vi "Divide XY (multiple).vi"(8 "error in (no error)":errorcluster, 9 "y":cluster{"X-array":dbl[], "Y-array":dbl[]}, 11 "XY-data":cluster{"X-array":dbl[], "Y-array":dbl[]}[](array[cluster]) {"Y-array" format="%.2p"; "X-array" format="%.2p"}) -> (0 "error out":errorcluster, 3 "XY-data out":cluster{"X-array":dbl[], "Y-array":dbl[]}[](array[cluster]) {"Y-array" format="%.2p"; "X-array" format="%.2p"})   [LabVIEW 2019, in "xy_utilities.lvlib"]
doc: "Divide <b>y</b>'s y array by the y array of <b>XY-data</b>.\n\nWire data to the data input to determine the polymorphic instance to use or manually select the instance."
uses:
  xy_utilities.lvlib
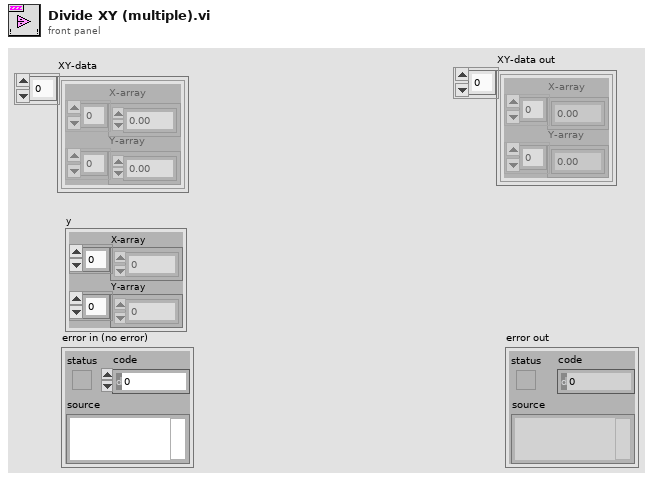
[diagram p1: front panel]
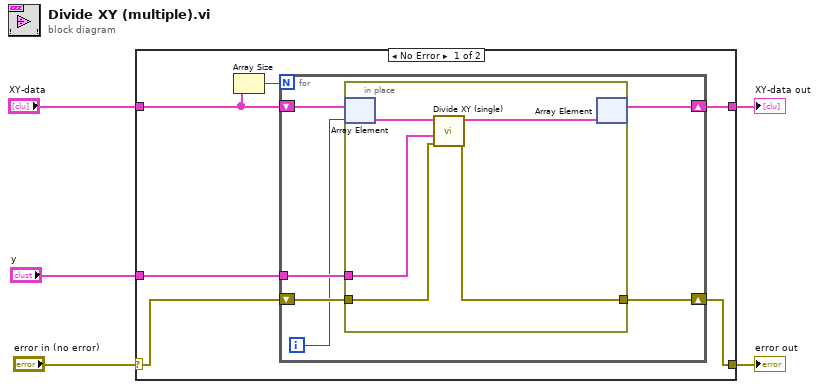
[diagram p0: block diagram]
diagram:
  n1 = case shown="No Error" "error in (no error)" {
    selector: "error in (no error)" -> [w9 w23]
    tunnel: [w8 w23] -> w1
    tunnel: "XY-data" -> [w6 w24]
    tunnel: [w11 w24] -> w3
    tunnel: "y" -> [w10 _]
    frame No Error {
      n2 = Array Size(array=w6) -> (size(s)=w7:i32)
      n3 = for {
        N: w7 -> [_]
        tunnel: w10 -> [w17]
        shift-right: [w15] -> w8
        shift-left: w9 -> [w16]
        shift-right: [w13] -> w11
        shift-left: w6 -> [w14]
        i -> [w12]
        n4 = in-place {
          in-place-border: w17 -> [w22]
          in-place-border: w16 -> [w21]
          in-place-border: [w20] -> w15
          n5 = in-place-array #1(w14, w12) -> (w19:cluster{"X-array":dbl[], "Y-array":dbl[]})
          n6 = call "Divide XY (single).vi"("error in (no error)"=w21, "y"=w22, "XY-data"=w19) -> ("error out"=w20:errorcluster, "XY-data out"=w18:cluster{"X-array":dbl[], "Y-array":dbl[]})  [unwired: 7 in]
          n7 = in-place-array #1(w18) -> (w13:cluster{"X-array":dbl[], "Y-array":dbl[]}[])  [unwired: 1 out]
        }
      }
    }
    frame Error {
    }
  }
  "error out" <- w1
  "XY-data out" <- w3
